vi "AlliGator Load FLI Dataset.vi"(5 "Image Type":string, 7 "Dataset Control References":T1, 8 "error in":errorcluster, 9 "Single Data Point Path":path, 10 "FLI Dataset Type":T2, 11 "AlliGator IV DVR in":refnum<data-value>) -> (0 "error out":errorcluster, 1 "File Path out":path, 3 "AlliGator IV DVR out":refnum<data-value>, 4 "Message":string)   [LabVIEW 2021, in "AlliGator Files.lvlib"]
doc: "Loads dataset of any kind, linking preparatory steps to the core VI."
uses:
  AlliGator Files.lvlib
  AlliGator FLI Dataset Type.ctl
  Internal Variables/AlliGator Internal Variables v2.ctl
  <vilib>/vision/Image Controls.llb/IMAQ Image.ctl
  Internal Variables/AlliGator Gate Image Set.ctl
  AlliGator Data Series Type.ctl
  Dual-Channel Datasets/AlliGator Dataset Channel.ctl
  Settings/AlliGator Gate Arithmetic.ctl
  Source Image/AlliGator Displayed Image.ctl
  Image/Named ROI Description.ctl
  Phasor Graph/AlliGator Decay Metadata v3.ctl
  Decay Analysis/Decay Preprocessing/AlliGator Decay Background Subtraction Info.ctl
  Decay Analysis/Decay Preprocessing/AlliGator Baseline Subtraction Method.ctl
  Graphs/XY Graph/XY Graph Plot Shift Parameters.ctl
  Graphs/XY Graph/XY Graph Plot Shift Method.ctl
  Decay Analysis/Decay Preprocessing/AlliGator Decay Extrapolation Parameters.ctl
  Phasor/Calibration Phasor (m, phi).ctl
  Phasor/Phasor Reference Series.ctl
  Phasor/Phasor Calibration Map v2.ctl
  Phasor/Phasor (g, s).ctl
  Phasor Graph/AlliGator Raw Phasor Plot Data v4.ctl
  Phasor/Phasor Standard Deviation Options.ctl
  Phasor Plot/AlliGator Phasor Multi-Harmonic Data.ctl
  Phasor/Phasor Harmonic Data.ctl
  Decay Fit Parameter Map/AlliGator Decay Fit Options & Parameters v2.ctl
  Fits/IRF(X)PSED/Decay Fit Options v2.ctl
  Fits/Decay Convolution/Decay Model.ctl
  Fits/Residual Type.ctl
  Fits/IRF(X)PSED/Fit Weights Type.ctl
  Fits/Non-linear Fitting Method v2.ctl
  Fits/Fit Calculation Method.ctl
  Fits/Non-linear Fitting Algorithm.ctl
  Decay Analysis/Decay Fit/AlliGator Decay Fit Parameter Constraints 2.ctl
  Fits/IRF(X)PSED/Decay Fit Parameters In List.ctl
  Fits/IRF(X)PSED/MLE Baseline Offset Type.ctl
  Decay Analysis/Decay Preprocessing/AlliGator Decay Preprocessing Parameters.ctl
  Fits/IRF(X)PSED/Decay Fit Parameters & Derived Quantities List v2.ctl
  Decay Fit Parameter Map/AlliGator Parameter Maps Data.ctl
  GUI/AlliGator Dataset Ctrl Refnums.ctl
  <vilib>/Utility/error.llb/Error Cluster From Error Code.vi
  <vilib>/ErrorRing/Error Ring.xnode
  Becker-Hickl Files/Becker-Hickl Files.lvlib
  PicoQuant/PicoQuant.lvlib
  HDF5/AlliGator HDF5.lvlib
  Phasor/Phasor.lvlib
  Image/Image.lvlib
  Decay Analysis/Decay Preprocessing/AlliGator Decay Preprocessing.lvlib
  Graphs/XY Graph/XY Graph Add-Ons.lvlib
  Phasor Graph/AlliGator Phasor Graph.lvlib
  Internal Variables/AlliGator Internal Variables.lvlib
  Phasor Plot/AlliGator Phasor Plot.lvlib
  Source Image/AlliGator Source Image.lvlib
  Fits/Fits.lvlib
  Decay Analysis/Decay Fit/AlliGator Decay Fit.lvlib
  Decay Fit Parameter Map/AlliGator Decay Fit Parameter Map.lvlib
  Settings/AlliGator Settings.lvlib
  GUI/AlliGator GUI.lvlib
  Dual-Channel Datasets/AlliGator Dual-Channel Datasets.lvlib
panel:
  # "see the AlliGator License on the block diagram (Ctrl+E or Window:Show Block Diagram)"
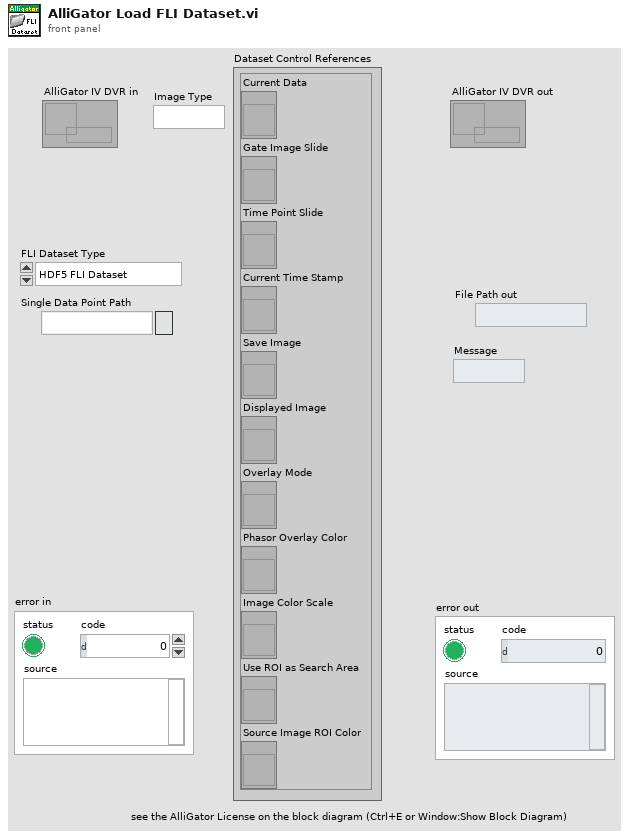
[diagram p1: front panel]
types:
  T1 = typedef "AlliGator GUI.lvlib/AlliGator Dataset Ctrl Refnums.ctl" = cluster{"Current Data":refnum<vi>, "Gate Image Slide":refnum<vi>, "Time Point Slide":refnum<vi>, "Current Time Stamp":refnum<vi>, "Save Image":refnum<vi>, "Displayed Image":refnum<vi>, "Overlay Mode":refnum<vi>, "Phasor Overlay Color":refnum<vi>, "Image Color Scale":refnum<vi>, "Use ROI as Search Area":refnum<vi>, "Source Image ROI Color":refnum<vi>}
  T2 = typedef "AlliGator Files.lvlib/AlliGator FLI Dataset Type.ctl" = enum16{"HDF5 FLI Dataset", "Gate Image Folder", ".sdt FLI Dataset (Becker & Hickl)", ".ptu FLI Dataset (PicoQuant)", "SS1 FLI Dataset", "SS2 FLI Dataset", "I/m/phi Dataset", ".bin FLI Dataset (PicoQuant Binned)", ".bin FLI Dataset (Piccolo Binned)", ".mat FLI Dataset"}
  T3 = typedef "AlliGator HDF5.lvlib/AlliGator FLI Data File Information.ctl" = cluster{"Load Single Gate Image VI Refnum":refnum<vi>, "File Info":variant, "FLI Parameters":T4, "FLI Dataset Type":T2}
  T4 = typedef "Phasor.lvlib/Phasor Fluorescence Lifetime Parameters v3.ctl" = cluster{"# Pixel X":i32, "# Pixel Y":i32, "# Gates":i32, "# Datasets":i32, "Gate Image Exposure":dbl[unit], "Macrotime Gate Separation":dbl[unit], "Nanotime Gate Separation":dbl[unit], "Gate Width":dbl[unit], "Laser Period":dbl[unit], "SYNC Period":dbl[unit], "Gate Image Integration":dbl[unit]}
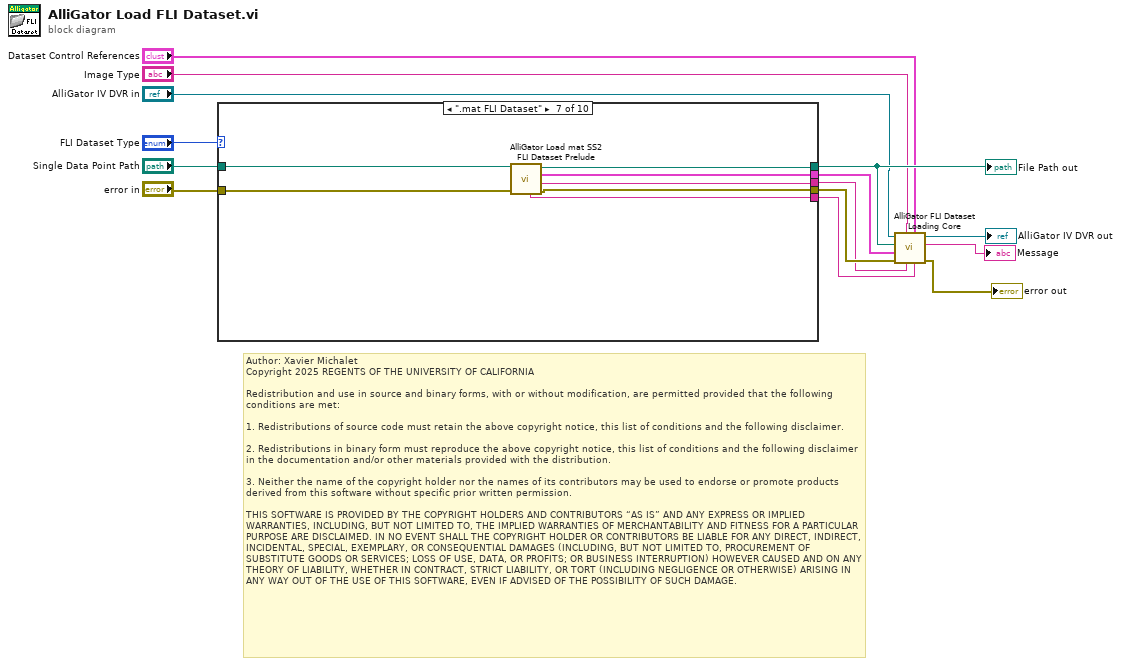
[diagram p0: block diagram]
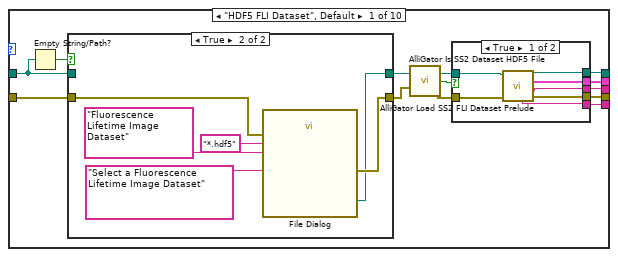
[diagram p2: hidden frame]
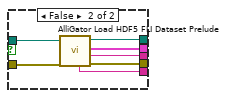
[diagram p4: hidden frame]
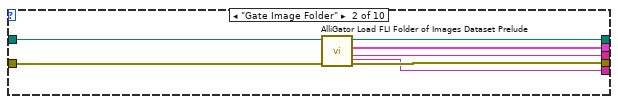
[diagram p5: hidden frame]
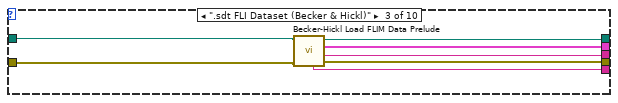
[diagram p6: hidden frame]
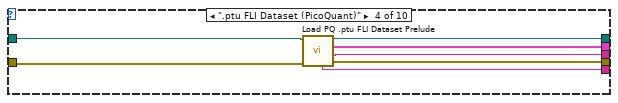
[diagram p7: hidden frame]
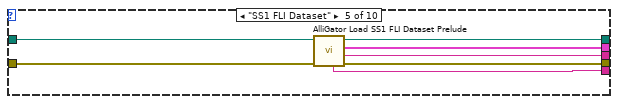
[diagram p8: hidden frame]
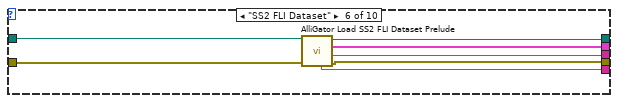
[diagram p9: hidden frame]
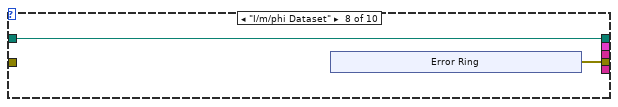
[diagram p10: hidden frame]
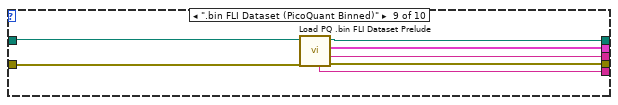
[diagram p11: hidden frame]
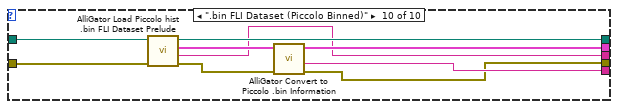
[diagram p12: hidden frame]
diagram:
  # "Author: Xavier Michalet\nCopyright 2025 REGENTS OF THE UNIVERSITY OF CALIFORNIA\n\nRedistribution and use in source and binary forms, with or without modification, are permitted provided that the following conditions are met:\n\n1. Redistributions of source code must retain the above copyright notice, this list of conditions and the following disclaimer.\n\n2. Redistributions in binary form must reproduce the above copyright notice, this list of conditions and the following disclaimer in the documentation and/or other materials provided with the distribution.\n\n3. Neither the name of the copyright holder nor the names of its contributors may be used to endorse or promote products derived from this software without specific prior written permission.\n\nTHIS SOFTWARE IS PROVIDED BY THE COPYRIGHT HOLDERS AND CONTRIBUTORS “AS IS” AND ANY EXPRESS OR IMPLIED WARRANTIES, INCLUDING, BUT NOT LIMITED TO, THE IMPLIED WARRANTIES OF MERCHANTABILITY AND FITNESS FOR A PARTICULAR PURPOSE ARE DISCLAIMED. IN NO EVENT SHALL THE COPYRIGHT HOLDER OR CONTRIBUTORS BE LIABLE FOR ANY DIRECT, INDIRECT, INCIDENTAL, SPECIAL, EXEMPLARY, OR CONSEQUENTIAL DAMAGES (INCLUDING, BUT NOT LIMITED TO, PROCUREMENT OF SUBSTITUTE GOODS OR SERVICES; LOSS OF USE, DATA, OR PROFITS; OR BUSINESS INTERRUPTION) HOWEVER CAUSED AND ON ANY THEORY OF LIABILITY, WHETHER IN CONTRACT, STRICT LIABILITY, OR TORT (INCLUDING NEGLIGENCE OR OTHERWISE) ARISING IN ANY WAY OUT OF THE USE OF THIS SOFTWARE, EVEN IF ADVISED OF THE POSSIBILITY OF SUCH DAMAGE."
  n1 = case shown="\".mat FLI Dataset\"" "FLI Dataset Type" {
    tunnel: [w26 w50 w57 w64 w76 w78 w85 w92 w102 w104] -> w5
    tunnel: [w22 w53 w60 w67 w75 w81 w88 w91 w98 w111] -> w12
    tunnel: [w23 w52 w59 w66 w74 w80 w87 _ w99 w107] -> w13
    tunnel: [w24 w51 w58 w65 w73 w79 w86 _ w100 w106] -> w4
    tunnel: [w25 w49 w56 w63 w72 w77 w84 _ w101 w105] -> w3
    tunnel: "Single Data Point Path" -> [w15 w54 w61 w69 w71 w83 w90 w91 w97 w110]
    tunnel: "error in" -> [w18 w55 w62 w68 w70 w82 w89 _ w103 w112]
    frame "HDF5 FLI Dataset", Default {
      n2 = Empty String/Path?(string/path=w15) -> (empty?=w19:bool)
      n3 = case shown="True" w19 {
        tunnel: w18 -> [w28 w31]
        tunnel: [w28 w30] -> w17
        tunnel: [w27 w29] -> w16
        tunnel: w15 -> [w27 _]
        frame False {
        }
        frame True {
          n4 = call "File Dialog"("prompt"="Select a Fluorescence Lifetime Image Dataset", "error in"=w31, "pattern (all files)"="*.hdf5", "pattern label"="Fluorescence Lifetime Image Dataset") -> ("selected path"=w29:path, "error out"=w30:errorcluster)  [unwired: 8 in, 2 out]
        }
      }
      n5 = call "AlliGator Is SS2 Dataset HDF5 File.vi"("File Path"=w16, "Error In"=w17) -> ("Is SS2 Dataset?"=w20:bool, "Error Out"=w21:errorcluster)  [unwired: 12 in]
      n6 = case shown="True" w20 {
        tunnel: w21 -> [w41 w48]
        tunnel: [w39 w47] -> w26
        tunnel: [w38 w46] -> w25
        tunnel: [w37 w45] -> w24
        tunnel: [w36 w44] -> w23
        tunnel: [w40 w43] -> w22
        tunnel: w16 -> [w35 w42]
        frame True {
          n7 = call "AlliGator Load SS2 FLI Dataset Prelude.vi"("error in (no error)"=w41, "File Path in"=w35) -> ("error out"=w39:errorcluster, "Metadata"=w37:string, "FLI Data File Information"=w36:T3, "File Path out"=w40:path, "Data Description"=w38:string)  [unwired: 5 in]
        }
        frame False {
          n8 = call "AlliGator Load HDF5 FLI Dataset Prelude.vi"("error in (no error)"=w48, "File Path"=w42) -> ("error out"=w47:errorcluster, "Metadata"=w45:string, "FLI Data File Information"=w44:T3, "File Path out"=w43:path, "Data Description"=w46:string)  [unwired: 5 in]
        }
      }
    }
    frame "Gate Image Folder" {
      n9 = call "AlliGator Load FLI Folder of Images Dataset Prelude.vi"("error in (no error)"=w55, "Folder Path in"=w54) -> ("error out"=w50:errorcluster, "Metadata"=w51:string, "FLI Data File Information"=w52:T3, "Folder Path out"=w53:path, "Data Description"=w49:string)  [unwired: 5 in]
    }
    frame ".sdt FLI Dataset (Becker & Hickl)" {
      n10 = call "Becker-Hickl Load FLIM Data Prelude.vi"("error in (no error)"=w62, "File Path in"=w61) -> ("error out"=w57:errorcluster, "Metadata"=w58:string, "FLI Data File Information"=w59:T3, "File Path out"=w60:path, "Data Description"=w56:string)  [unwired: 5 in]
    }
    frame ".ptu FLI Dataset (PicoQuant)" {
      n11 = call "Load PQ .ptu FLI Dataset Prelude.vi"("error in (no error)"=w68, "File Path in"=w69) -> ("error out"=w64:errorcluster, "Metadata"=w65:string, "FLI Data File Information"=w66:T3, "File Path out"=w67:path, "Data Description"=w63:string)  [unwired: 5 in]
    }
    frame "SS1 FLI Dataset" {
      n12 = call "AlliGator Load SS1 FLI Dataset Prelude.vi"("error in (no error)"=w70, "Path in"=w71) -> ("error out"=w76:errorcluster, "Metadata"=w73:string, "FLI Data File Information"=w74:T3, "Path out"=w75:path, "Data Description"=w72:string)  [unwired: 5 in]
    }
    frame "SS2 FLI Dataset" {
      n13 = call "AlliGator Load SS2 FLI Dataset Prelude.vi"("error in (no error)"=w82, "File Path in"=w83) -> ("error out"=w78:errorcluster, "Metadata"=w79:string, "FLI Data File Information"=w80:T3, "File Path out"=w81:path, "Data Description"=w77:string)  [unwired: 5 in]
    }
    frame ".mat FLI Dataset" {
      n14 = call "AlliGator Load mat SS2 FLI Dataset Prelude.vi"("error in (no error)"=w89, "File Path in"=w90) -> ("error out"=w85:errorcluster, "Metadata"=w86:string, "FLI Data File Information"=w87:T3, "File Path out"=w88:path, "Data Description"=w84:string)  [unwired: 5 in]
    }
    frame "I/m/phi Dataset" {
      n15 = xnode "Error Ring"() -> ("error out"=w92:errorcluster)
    }
    frame ".bin FLI Dataset (PicoQuant Binned)" {
      n16 = call "Load PQ .bin FLI Dataset Prelude.vi"("error in (no error)"=w103, "File Path in"=w97) -> ("error out"=w102:errorcluster, "Metdata"=w100:string, "FLI Data File Information"=w99:T3, "File Path out"=w98:path, "Data Description"=w101:string)  [unwired: 5 in]
    }
    frame ".bin FLI Dataset (Piccolo Binned)" {
      n17 = call "AlliGator Load Piccolo hist .bin FLI Dataset Prelude.vi"("error in (no error)"=w112, "File Path in"=w110) -> ("error out"=w109:errorcluster, "Metdata"=w106:string, "FLI Data File Information"=w108:T3, "File Path out"=w111:path)  [unwired: 5 in, 1 out]
      n18 = call "AlliGator Convert to Piccolo .bin Information.vi"("error in (no error)"=w109, "FLI Data File Information in"=w108) -> ("error out"=w104:errorcluster, "Data Description out"=w105:string, "FLI Data File Information out"=w107:T3)  [unwired: 7 in]
    }
  }
  "File Path out" <- w12
  n19 = call "AlliGator FLI Dataset Loading Core.vi"("Data Description"=w3, "Control References"="Dataset Control References", "Metadata"=w4, "Image Type"="Image Type", "error in (no error)"=w5, "FLI Data File Information"=w13, "selected path"=w12, "Data Value Reference in"="AlliGator IV DVR in") -> ("error out"=→"error out":errorcluster, "Message"=→"Message":string, "Data Value Reference out"=→"AlliGator IV DVR out":refnum<data-value>)  [unwired: 1 in]
